vi "Flags.vi"() -> ()   [LabVIEW 2012]
panel:
  out "done":bool
  # "a global done variable that all the visible subVIs monitor - if it is flagged, all the subVIs flag a local done, which shuts itself down (\"value signaling\"is used, which simulates user input and can trigger an event and even structures are used heavily throughout all of the programs - this is why a local variable needs to be signaled, because you cannot value signal a global variable)"
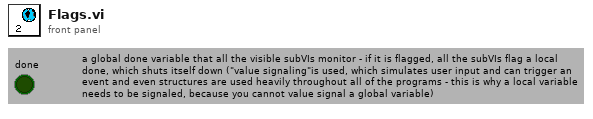
[diagram p1: front panel]
diagram:
